vi "ROI_to_string.vi"(10 "ROI Parameters":T1) -> (2 "String":string)   [LabVIEW 2016]
uses:
  Controls/ScanParameters/ROI_set.ctl
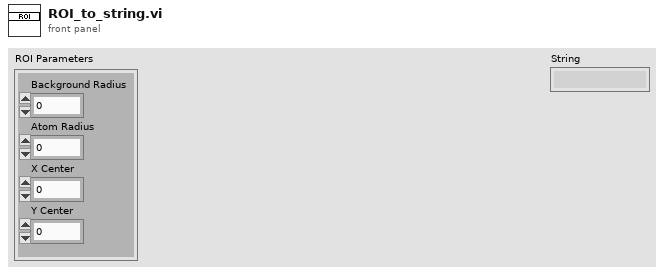
[diagram p1: front panel]
types:
  T1 = typedef "ROI_set.ctl" = cluster{"Background Radius":dbl, "Atom Radius":dbl, "X Center":dbl, "Y Center":dbl}
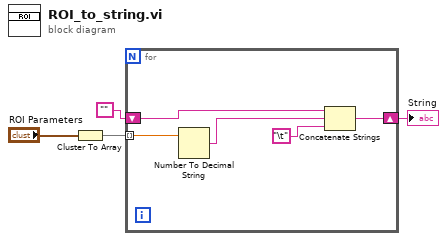
[diagram p0: block diagram]
diagram:
  n1 = Cluster To Array(cluster="ROI Parameters") -> (array=w3:dbl[])
  n2 = for {
    tunnel: w3 -> [w9] mode=indexing
    shift-right: [w6] -> w1
    shift-left: "" -> [w7]
    n3 = Number To Decimal String(number=w9) -> (decimal integer string=w8:string)  [unwired: 1 in]
    n4 = Concatenate Strings(w7, w8, "\t") -> (w6:string)
  }
  "String" <- w1
